vi "Test Load Unicode Paths.vi"(8 "error in (no error)":errorcluster) -> (0 "error out":errorcluster, 3 "Pass?":bool)   [LabVIEW 2020]
uses:
  G-Image/Image IO/Polymorphic VIs/Load SVG Image (UTF-8 Path).vi
  G-Image/Image IO/Polymorphic VIs/Load Image (UTF-8 Path).vi
  G-Image/G-Image.lvlib
panel:
  out "Array":cluster{string, "new picture":picture}[](array[cluster])
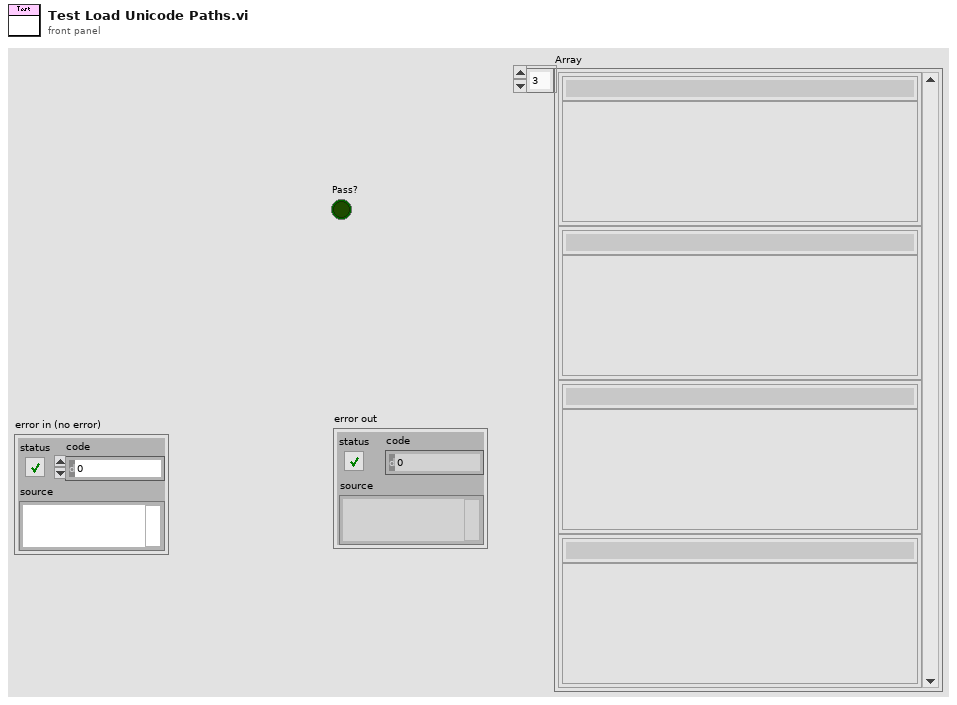
[diagram p1: front panel]
types:
  T1 = typedef "imagedata.ctl" = cluster{"image type":i32, "image depth":i32, "image":u8[], "mask":u8[], "colors":u32[], "Rectangle":cluster{"left":i16, "top":i16, "right":i16, "bottom":i16}}
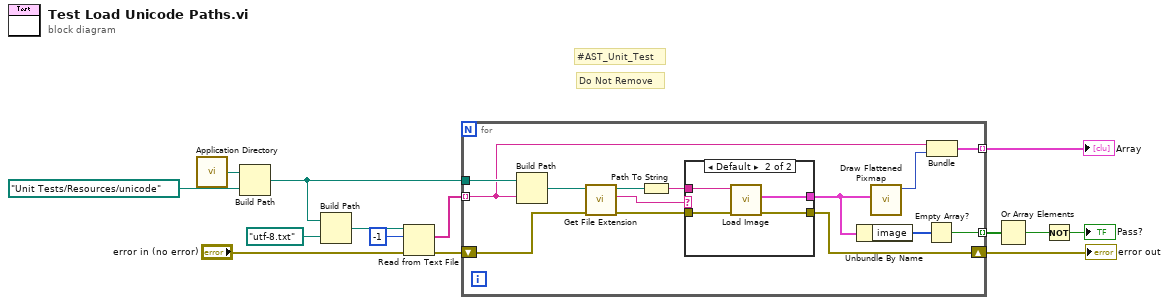
[diagram p0: block diagram]
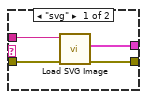
[diagram p2: hidden frame]
diagram:
  # "Do Not Remove"
  # "#AST_Unit_Test"
  n1 = call <vilib>:"Application Directory.vi"() -> ("Application Directory"=w12:path)
  n2 = Build Path(base path=w12, name or relative path=path "Unit Tests/Resources/unicode" ("Path")) -> (appended path=w6:path)
  n3 = Build Path(base path=w6, name or relative path=path "utf-8.txt") -> (appended path=w9:path)
  n4 = Read from Text File(file (use dialog)=w9, count=-1 ("count (1)"), error in="error in (no error)") -> (text=w7:string[], error out=w4:errorcluster)  [unwired: 1 in, 2 out]
  n5 = for {
    shift-right: [w25] -> w14
    shift-left: w4 -> [w24]
    tunnel: [w28] -> w13 mode=indexing
    tunnel: w7 -> [w19] mode=indexing
    tunnel: w6 -> [w26]
    tunnel: [w15] -> w3 mode=indexing
    n6 = Build Path(base path=w26, name or relative path=w19) -> (appended path=w23:path)
    n7 = call <vilib>:"Get File Extension.vi"("error in (no error)"=w24, "file"=w23) -> ("error out"=w20:errorcluster, "lowercase file extension"=w21:string, "dup file"=w22:path)  [unwired: 5 in, 2 out]
    n8 = Path To String(path=w22) -> (string=w27:string)
    n9 = case shown="Default" w21 {
      tunnel: w27 -> [w32 w36]
      tunnel: [w31 w35] -> w17
      tunnel: w20 -> [w30 w34]
      tunnel: [w29 w33] -> w25
      frame "svg" {
        n10 = call-poly "Load SVG Image.vi"("error in (no error)"=w30, "Path In"=w32) -> ("error out"=w29:errorcluster, "Image"=w31:T1)  [unwired: 7 in, 1 out]
      }
      frame Default {
        n11 = call-poly "Load Image.vi"("error in (no error)"=w34, "Path In"=w36) -> ("error out"=w33:errorcluster, "Image"=w35:T1)  [unwired: 7 in, 1 out]
      }
    }
    n12 = Unbundle By Name(w17) -> ("image"=w16:u8[])
    n13 = call <vilib>:"Draw Flattened Pixmap.vi"("image data"=w17) -> ("new picture"=w18:picture)  [unwired: 8 in]
    n14 = Empty Array?(array=w16) -> (empty?=w15:bool)
    n15 = Bundle(w19, "new picture"=w18) -> (w28:cluster{string, "new picture":picture})  [unwired: 1 in]
  }
  "error out" <- w14
  "Array" <- w13
  n16 = Or Array Elements(Boolean array=w3) -> (logical OR=w2:bool)
  n17 = Not(x=w2) -> (.not. x?=→"Pass?":bool)
